vi "SERIAL_DecodeBinaryPacket.vi"(0 "navX DevRef":T1={"SerialPortRef"={"DevStatus"={"status"=FALSE, "code"=0, "source"=""}, "Serial Port Name"=""}, "Board Information"={"WhoAmI (50 | 0x32)"=0, "Board Revision"=0, "Firmware Major Version"=0, "Firmware Minor Version"=0, "NAVX_BOARD_CAPABILITY"={"OMNIMOUNT"=FALSE, "YAW_RESET"=FALSE, "VEL_AND_DISP"=FALSE}, "NAVX_BOARD_YAW_AXIS"={"BOARD_YAW_AXIS_UP"=FALSE, "BOARD_YAW_AXIS"=0}}, "Status"={"Update Rate Hz"=0, "Accelerometer Full-Scale Range"=0, "Gyro Full-Scale Range"=0, "NAVX_OP_STATUS"=0, "NAVX_CAL_STATUS"=0, "NAVX_SELFTEST_STATUS"=0, "NAVX_SENSOR_STATUS"={"MOVING"=FALSE, "YAW_STABLE"=FALSE, "MAG_DISTURBANCE"=FALSE, "ALTITUDE_VALID"=FALSE, "SEALEVEL_PRESS_SET"=FALSE, "FUSED_HEADING_VALID"=FALSE}}, "Offsets"={"Yaw"=0.0, "Quat W"=0.0, "Quat X"=0.0, "Quat Y"=0.0, "Quat Z"=0.0}, "Update Rate (4Hz-60Hz)"=50, "Nav6Mode (YPR)"=enum."YPR", "refnum name"="", "error"={"status"=FALSE, "code"=0, "source"=""}, "Loop VI Refnum"=refnum, "Serial Port"=enum."Onboard RS-232"} {"Status"."NAVX_OP_STATUS" items=["INITIALIZING", "SELFTEST_IN_PROGRESS", "ERROR", "IMU_AUTOCAL_IN_PROGRESS", "NORMAL"]; "Status"."NAVX_CAL_STATUS" items=["IMU_CAL_STATE_MASK"=3, "IMU_CAL_INPROGRESS"=0, "IMU_CAL_ACCUMULATE"=1, "IMU_CAL_COMPLETE"=2, "MAG_CAL_COMPLETE"=4, "BARO_CAL_COMPLETE"=8]}, 1 "PacketType":string, 2 "Buffer":string) -> (7 "navX DevRef":T1={"SerialPortRef"={"DevStatus"={"status"=FALSE, "code"=0, "source"=""}, "Serial Port Name"=""}, "Board Information"={"WhoAmI (50 | 0x32)"=0, "Board Revision"=0, "Firmware Major Version"=0, "Firmware Minor Version"=0, "NAVX_BOARD_CAPABILITY"={"OMNIMOUNT"=FALSE, "YAW_RESET"=FALSE, "VEL_AND_DISP"=FALSE}, "NAVX_BOARD_YAW_AXIS"={"BOARD_YAW_AXIS_UP"=FALSE, "BOARD_YAW_AXIS"=0}}, "Status"={"Update Rate Hz"=0, "Accelerometer Full-Scale Range"=0, "Gyro Full-Scale Range"=0, "NAVX_OP_STATUS"=0, "NAVX_CAL_STATUS"=0, "NAVX_SELFTEST_STATUS"=0, "NAVX_SENSOR_STATUS"={"MOVING"=FALSE, "YAW_STABLE"=FALSE, "MAG_DISTURBANCE"=FALSE, "ALTITUDE_VALID"=FALSE, "SEALEVEL_PRESS_SET"=FALSE, "FUSED_HEADING_VALID"=FALSE}}, "Offsets"={"Yaw"=0.0, "Quat W"=0.0, "Quat X"=0.0, "Quat Y"=0.0, "Quat Z"=0.0}, "Update Rate (4Hz-60Hz)"=50, "Nav6Mode (YPR)"=enum."YPR", "refnum name"="", "error"={"status"=FALSE, "code"=0, "source"=""}, "Loop VI Refnum"=refnum, "Serial Port"=enum."Onboard RS-232"} {"Status"."NAVX_OP_STATUS" items=["INITIALIZING", "SELFTEST_IN_PROGRESS", "ERROR", "IMU_AUTOCAL_IN_PROGRESS", "NORMAL"]; "Status"."NAVX_CAL_STATUS" items=["IMU_CAL_STATE_MASK"=3, "IMU_CAL_INPROGRESS"=0, "IMU_CAL_ACCUMULATE"=1, "IMU_CAL_COMPLETE"=2, "MAG_CAL_COMPLETE"=4, "BARO_CAL_COMPLETE"=8]})   [LabVIEW 2014, in "navX-MXP IMU.lvlib"]
uses:
  navX-MXP IMU.lvlib
  COMMON/TypeDefs/Data TypeDefs/navX Board Information.ctl
  COMMON/TypeDefs/Value TypeDefs/navX NAVX_BOARD_CAPABILITY.ctl
  COMMON/TypeDefs/Value TypeDefs/navX NAVX_BOARD_YAW_AXIS.ctl
  navX Serial DevRef.ctl
  <vilib>/Rock Robotics/WPI/SerialPort/WPI_SerialPortRef.ctl
  COMMON/TypeDefs/Data TypeDefs/navX Status Data.ctl
  COMMON/TypeDefs/Value TypeDefs/navX NAVX_OP_STATUS.ctl
  COMMON/TypeDefs/Value TypeDefs/navX NAVX_CAL_STATUS.ctl
  COMMON/TypeDefs/Value TypeDefs/navX NAVX_SENSOR_STATUS.ctl
  TypeDefs/navX Serial Mode.ctl
  IO/NI WPI/WPI_SerialPort_USB.ctl
  COMMON/TypeDefs/Data TypeDefs/navX YPRH Data.ctl
  COMMON/TypeDefs/Data TypeDefs/navX Vector Data.ctl
  COMMON/TypeDefs/Data TypeDefs/navX Quaternion Data.ctl
panel:
  out "Valid? 2":bool
  out "Valid?":bool
  in  "Board Information":T3
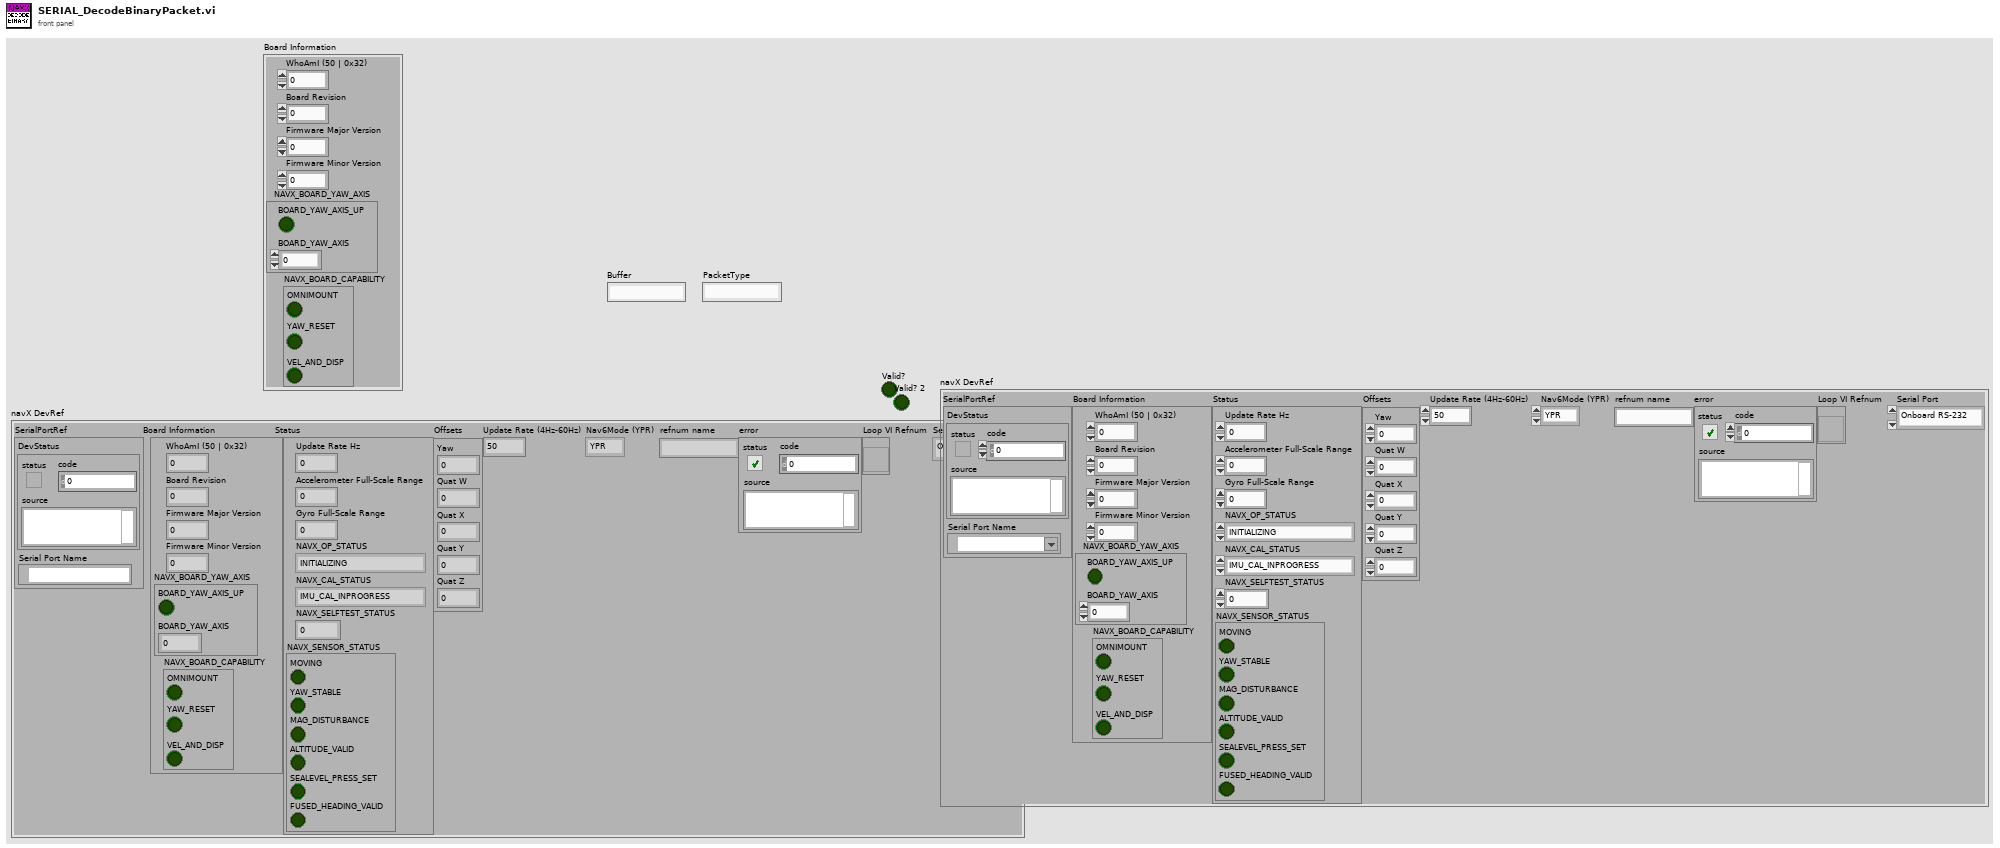
[diagram p1: front panel]
types:
  T1 = typedef "navX-MXP IMU.lvlib/navX Serial DevRef.ctl" = cluster{"SerialPortRef":T2, "Board Information":T3, "Status":T6, "Offsets":cluster{"Yaw":dbl, "Quat W":dbl, "Quat X":dbl, "Quat Y":dbl, "Quat Z":dbl}, "Update Rate (4Hz-60Hz)":u8, "Nav6Mode (YPR)":T10, "refnum name":string, "error":errorcluster, "Loop VI Refnum":refnum<vi>, "Serial Port":T11}
  T2 = typedef "WPI_SerialPortRef.ctl" = cluster{"DevStatus":errorcluster, "Serial Port Name":refnum<visa-resource-name>}
  T3 = typedef "navX-MXP IMU.lvlib/navX Board Information.ctl" = cluster{"WhoAmI (50 | 0x32)":u8, "Board Revision":u8, "Firmware Major Version":u8, "Firmware Minor Version":u8, "NAVX_BOARD_CAPABILITY":T4, "NAVX_BOARD_YAW_AXIS":T5}
  T4 = typedef "navX-MXP IMU.lvlib/navX NAVX_BOARD_CAPABILITY.ctl" = cluster{"OMNIMOUNT":bool, "YAW_RESET":bool, "VEL_AND_DISP":bool}
  T5 = typedef "navX-MXP IMU.lvlib/navX NAVX_BOARD_YAW_AXIS.ctl" = cluster{"BOARD_YAW_AXIS_UP":bool, "BOARD_YAW_AXIS":u8}
  T6 = typedef "navX-MXP IMU.lvlib/navX Status Data.ctl" = cluster{"Update Rate Hz":u8, "Accelerometer Full-Scale Range":u8, "Gyro Full-Scale Range":u16, "NAVX_OP_STATUS":T7, "NAVX_CAL_STATUS":T8, "NAVX_SELFTEST_STATUS":u8, "NAVX_SENSOR_STATUS":T9}
  T7 = typedef "navX-MXP IMU.lvlib/navX NAVX_OP_STATUS.ctl" = u8
  T8 = typedef "navX-MXP IMU.lvlib/navX NAVX_CAL_STATUS.ctl" = u8
  T9 = typedef "navX-MXP IMU.lvlib/navX NAVX_SENSOR_STATUS.ctl" = cluster{"MOVING":bool, "YAW_STABLE":bool, "MAG_DISTURBANCE":bool, "ALTITUDE_VALID":bool, "SEALEVEL_PRESS_SET":bool, "FUSED_HEADING_VALID":bool}
  T10 = typedef "navX-MXP IMU.lvlib/navX Serial Mode.ctl" = enum16{"YPR", "Gyro", "Quaternion", "AHRS", "AHRSPos"}
  T11 = typedef "navX-MXP IMU.lvlib/WPI_SerialPort_USB.ctl" = enum16{"Onboard RS-232", "MXP TTL", "USB"}
  T12 = typedef "navX-MXP IMU.lvlib/navX Quaternion Data.ctl" = cluster{"W":dbl, "X":dbl, "Y":dbl, "Z":dbl}
  T13 = typedef "navX-MXP IMU.lvlib/navX Vector Data.ctl" = cluster{"X":dbl, "Y":dbl, "Z":dbl}
  T14 = typedef "navX-MXP IMU.lvlib/navX YPRH Data.ctl" = cluster{"Yaw":dbl, "Pitch":dbl, "Roll":dbl, "Heading":dbl}
  T15 = cluster{"unsigned byte array[0]":u8, "unsigned byte array[1]":u8, "unsigned byte array[2]":u8, "unsigned byte array[3]":u8, "unsigned byte array[4]":u8, "unsigned byte array[5]":u8, "unsigned byte array[6]":u8, "unsigned byte array[7]":u8, "unsigned byte array[8]":u8}
  T16 = cluster{"[0]":u8, "[1]":u8, "[2]":u8, "[3]":u8, "[4]":u8, "[5]":u8, "[6]":u8, "[7]":u8, "[8]":u8}
  T17 = cluster{"Boolean array[0]":bool, "Boolean array[1]":bool, "Boolean array[2]":bool, "Boolean array[3]":bool, "Boolean array[4]":bool, "Boolean array[5]":bool}
  T18 = cluster{"[0]":dbl, "[1]":dbl, "[2]":dbl, "[3]":dbl}
  T19 = typedef "navX-MXP IMU.lvlib/navX AHRSPos Data.ctl" = cluster{"Quaternion":T12, "RawMag":T13, "CalMag":T13, "LinearAccel":T13, "Displacement":T13, "Velocity":T13, "Altitude":dbl, "FusedHeading":dbl, "MPU Temperature":dbl, "LastUpdateFPGATimestamp":dbl}
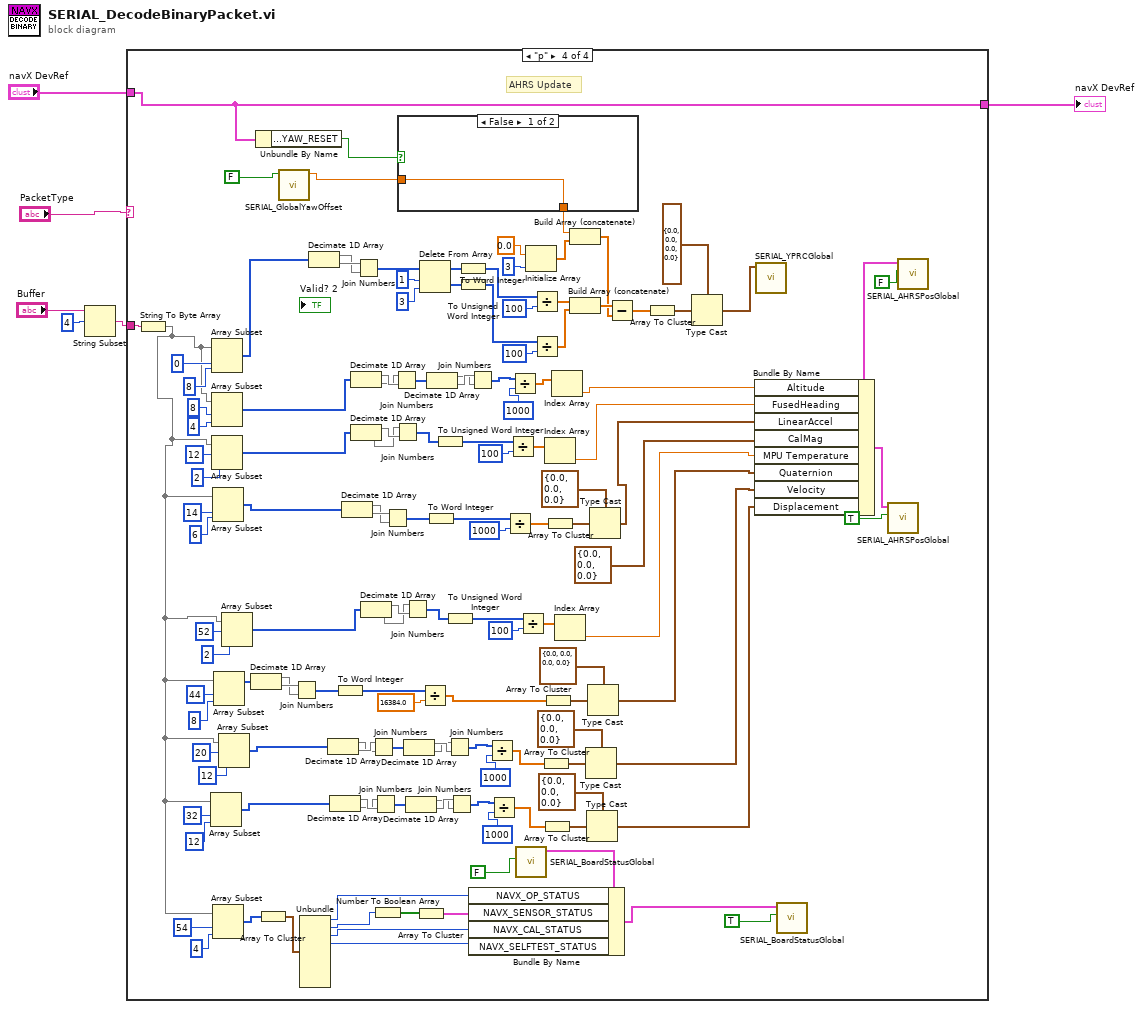
[diagram p0: block diagram]
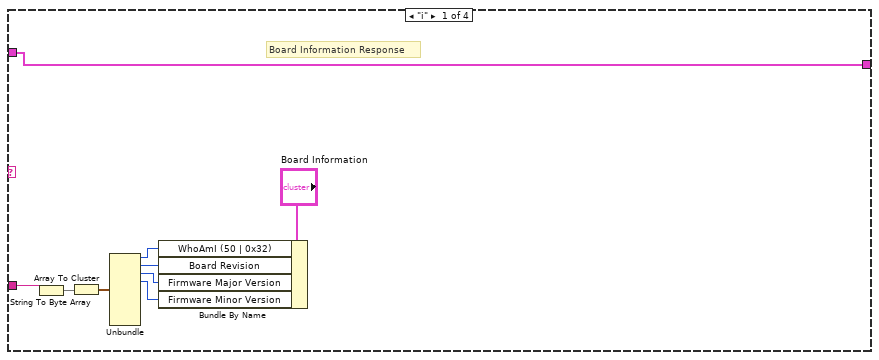
[diagram p2: hidden frame]
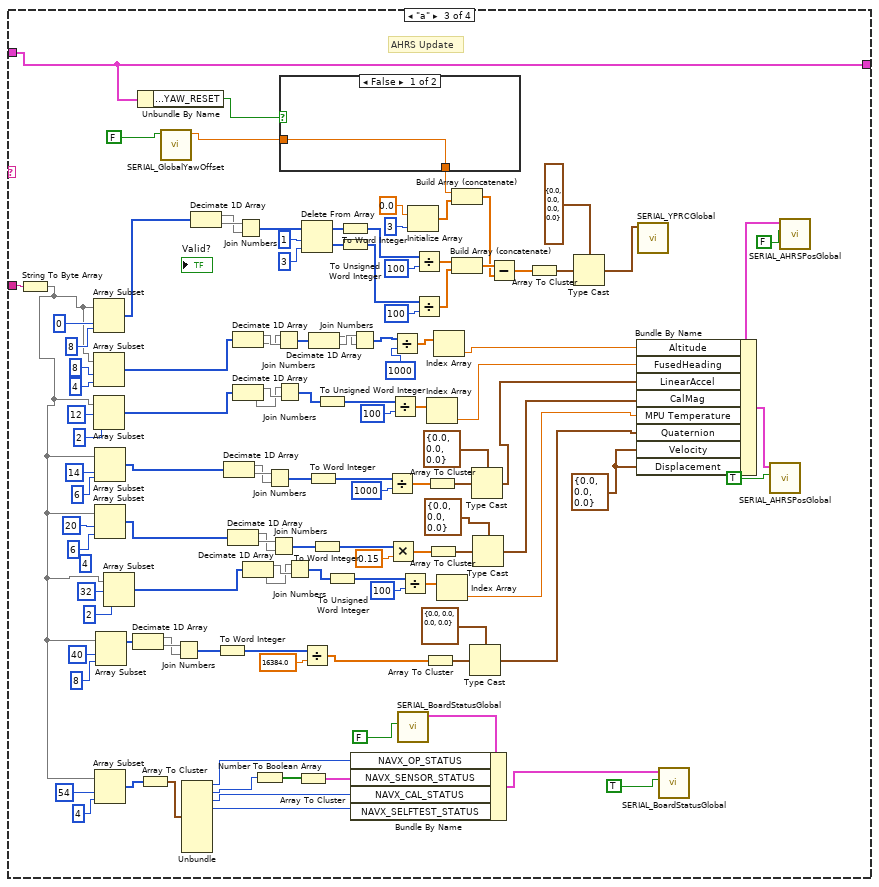
[diagram p4: hidden frame]
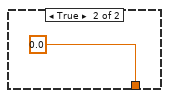
[diagram p5: hidden frame]
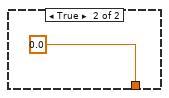
[diagram p6: hidden frame]
diagram:
  n1 = String Subset(string="Buffer", offset (0)=4) -> (substring=w4:string)  [unwired: 1 in]
  n2 = case shown="\"p\"" "PacketType" {
    tunnel: w4 -> [w9 _ w135 w272]
    tunnel: "navX DevRef" -> [w7 w16 w109 w246]
    tunnel: [w7 w16 w109 w246] -> w1
    frame "i" {
      # "Board Information Response"
      n3 = String To Byte Array(string=w9) -> (unsigned byte array=w8:u8[])
      n4 = Array To Cluster(array=w8) -> (cluster=w15:T15)
      n5 = Unbundle(w15) -> ("unsigned byte array[0]"=w13:u8, "unsigned byte array[1]"=w12:u8, "unsigned byte array[2]"=w11:u8, "unsigned byte array[3]"=w10:u8)  [unwired: 5 out]
      n6 = Bundle By Name(cluster="Board Information", "WhoAmI (50 | 0x32)"=w13, "Board Revision"=w12, "Firmware Major Version"=w11, "Firmware Minor Version"=w10) -> ()  [unwired: 1 out]
    }
    frame Default {
    }
    frame "a" {
      w18 = T13 {"X"=0.0, "Y"=0.0, "Z"=0.0} ("Vector")
      (unwired) 4
      # "AHRS Update"
      n7 = String To Byte Array(string=w135) -> (unsigned byte array=w22:u8[])
      n8 = Array Subset(array=w22, index=0, length=8) -> (w111:u8[])
      n9 = Array Subset(array=w22, index=8, length=4) -> (w89:u8[])
      n10 = Array Subset(array=w22, index=12, length=2) -> (w69:u8[])
      n11 = Array Subset(array=w22, index=14, length=6) -> (w56:u8[])
      n12 = Array Subset(array=w22, index=20, length=6) -> (w41:u8[])
      n13 = Array Subset(array=w22, index=54, length=4) -> (w100:u8[])
      n14 = Array Subset(array=w22, index=40, length=8) -> (w19:u8[])
      n15 = Array Subset(array=w22, index=32, length=2) -> (w40:u8[])
      n16 = Decimate 1D Array(w19) -> (w30:u8[], w31:u8[])
      n17 = Unbundle By Name(w109) -> ("Board Information.NAVX_BOARD_CAPABILITY.YAW_RESET"=w106:bool)
      n18 = Array To Cluster(array=w100) -> (cluster=w99:T16)
      n19 = call "SERIAL_GlobalYawOffset.vi"("Set"=FALSE) -> ("OutputYawOffset"=w107:dbl)  [unwired: 10 in]
      n20 = Join Numbers(hi=w31, lo=w30) -> ((hi.lo)=w29:u16[])
      n21 = Unbundle(w99) -> ("[0]"=w98:u8, "[1]"=w95:u8, "[2]"=w97:u8, "[3]"=w96:u8)  [unwired: 5 out]
      n22 = Decimate 1D Array(w111) -> (w133:u8[], w134:u8[])
      n23 = To Word Integer(number=w29) -> (16bit integer=w28:i16[])
      n24 = Decimate 1D Array(w56) -> (w64:u8[], w65:u8[])
      n25 = Decimate 1D Array(w41) -> (w52:u8[], w53:u8[])
      n26 = Decimate 1D Array(w89) -> (w88:u8[], w87:u8[])
      n27 = Decimate 1D Array(w69) -> (w68:u8[], w67:u8[])
      n28 = Join Numbers(hi=w134, lo=w133) -> ((hi.lo)=w131:u16[])
      n29 = Decimate 1D Array(w40) -> (w34:u8[], w33:u8[])
      n30 = Number To Boolean Array(number=w95) -> (Boolean array=w94:bool[])
      n31 = Join Numbers(hi=w65, lo=w64) -> ((hi.lo)=w63:u16[])
      n32 = Join Numbers(hi=w53, lo=w52) -> ((hi.lo)=w51:u16[])
      n33 = Join Numbers(hi=w87, lo=w88) -> ((hi.lo)=w86:u16[])
      n34 = Join Numbers(hi=w67, lo=w68) -> ((hi.lo)=w75:u16[])
      n35 = case shown="False" w106 {
        tunnel: w107 -> [w136 _]
        tunnel: [w136 0.0] -> w105
        frame False {
        }
        frame True {
        }
      }
      n36 = Join Numbers(hi=w33, lo=w34) -> ((hi.lo)=w35:u16[])
      n37 = Array To Cluster(array=w94) -> (cluster=w93:T17)
      n38 = Delete From Array(array=w131, length=1, index=3) -> (deleted portion=w127:u16[], array with subset deleted=w128:u16[])
      n39 = Divide(x=w28, y=16384.0) -> (x/y=w17:dbl[])
      n40 = To Word Integer(number=w63) -> (16bit integer=w62:i16[])
      n41 = Decimate 1D Array(w86) -> (w84:u16[], w85:u16[])
      n42 = To Word Integer(number=w51) -> (16bit integer=w50:i16[])
      n43 = To Unsigned Word Integer(number=w75) -> (unsigned 16bit integer=w74:u16[])
      n44 = To Unsigned Word Integer(number=w35) -> (unsigned 16bit integer=w36:u16[])
      n45 = To Word Integer(number=w128) -> (16bit integer=w114:i16[])
      n46 = To Unsigned Word Integer(number=w127) -> (unsigned 16bit integer=w126:u16[])
      n47 = Join Numbers(hi=w85, lo=w84) -> ((hi.lo)=w83:u32[])
      n48 = Divide(x=w62, y=1000) -> (x/y=w60:dbl[])
      n49 = Multiply(x=w50, y=0.15) -> (x*y=w49:dbl[])
      n50 = Divide(x=w74, y=100) -> (x/y=w72:dbl[])
      n51 = Divide(x=w83, y=i16 1000) -> (x/y=w81:dbl[])
      n52 = call "SERIAL_BoardStatusGlobal.vi"("Set"=FALSE) -> ("Status"=w101:T6)  [unwired: 9 in, 1 out]
      n53 = Bundle By Name(cluster=w101, "NAVX_OP_STATUS"=w98, "NAVX_SENSOR_STATUS"=w93, "NAVX_CAL_STATUS"=w97, "NAVX_SELFTEST_STATUS"=w96) -> (w91:T6)
      n54 = Divide(x=w36, y=100) -> (x/y=w38:dbl[])
      n55 = Initialize Array(0.0 ("element"), 3 ("dimension size")) -> (w120:dbl[])
      n56 = Divide(x=w114, y=i16 100) -> (x/y=w124:dbl[])
      n57 = Divide(x=w126, y=u16 100) -> (x/y=w123:dbl[])
      n58 = Array To Cluster(array=w17) -> (cluster=w26:T18)
      n59 = Index Array(array=w72) -> (element=w66:dbl)  [unwired: 1 in]
      n60 = Array To Cluster(array=w60) -> (cluster=w59:cluster{"[0]":dbl, "[1]":dbl, "[2]":dbl})
      n61 = Array To Cluster(array=w49) -> (cluster=w47:cluster{"[0]":dbl, "[1]":dbl, "[2]":dbl})
      n62 = Index Array(array=w81) -> (element=w76:dbl)  [unwired: 1 in]
      n63 = Index Array(array=w38) -> (element=w32:dbl)  [unwired: 1 in]
      n64 = Build Array (concatenate)(w105, w120) -> (w118:dbl[])
      n65 = Build Array (concatenate)(w124, w123) -> (w119:dbl[])
      n66 = Type Cast(type=T12 {"W"=0.0, "X"=0.0, "Y"=0.0, "Z"=0.0} ("Quaternion"), x=w26) -> (*(type *) &x=w24:T12)
      n67 = Type Cast(type=T13 {"X"=0.0, "Y"=0.0, "Z"=0.0} ("Vector"), x=w59) -> (*(type *) &x=w54:T13)
      n68 = Type Cast(type=T13 {"X"=0.0, "Y"=0.0, "Z"=0.0} ("Vector"), x=w47) -> (*(type *) &x=w45:T13)
      n69 = Subtract(x=w119, y=w118) -> (x-y=w117:dbl[])
      n70 = Array To Cluster(array=w117) -> (cluster=w116:T18)
      n71 = Type Cast(type=T14 {"Yaw"=0.0, "Pitch"=0.0, "Roll"=0.0, "Heading"=0.0} ("YPRH"), x=w116) -> (*(type *) &x=w110:T14)
      n72 = call "SERIAL_YPRCGlobal.vi"("YPRH"=w110) -> ()  [unwired: 9 in, 2 out]
      n73 = call "SERIAL_BoardStatusGlobal.vi"("Set"=TRUE, "Status"=w91) -> ()  [unwired: 8 in, 2 out]
      n74 = call "SERIAL_AHRSPosGlobal.vi"("Set"=FALSE) -> ("AHRSPos Data"=w79:T19)  [unwired: 10 in]
      n75 = Bundle By Name(cluster=w79, "Altitude"=w76, "FusedHeading"=w66, "LinearAccel"=w54, "CalMag"=w45, "MPU Temperature"=w32, "Quaternion"=w24, "Velocity"=w18, "Displacement"=w18) -> (w77:T19)
      n76 = call "SERIAL_AHRSPosGlobal.vi"("Set"=TRUE, "AHRSPos Data"=w77) -> ()  [unwired: 9 in, 1 out]
    }
    frame "p" {
      # "AHRS Update"
      n77 = String To Byte Array(string=w272) -> (unsigned byte array=w163:u8[])
      n78 = Array Subset(array=w163, index=32, length=12) -> (w147:u8[])
      n79 = Array Subset(array=w163, index=0, length=8) -> (w248:u8[])
      n80 = Array Subset(array=w163, index=8, length=4) -> (w226:u8[])
      n81 = Array Subset(array=w163, index=12, length=2) -> (w206:u8[])
      n82 = Array Subset(array=w163, index=14, length=6) -> (w193:u8[])
      n83 = Array Subset(array=w163, index=54, length=4) -> (w237:u8[])
      n84 = Array Subset(array=w163, index=44, length=8) -> (w169:u8[])
      n85 = Array Subset(array=w163, index=20, length=12) -> (w146:u8[])
      n86 = Array Subset(array=w163, index=52, length=2) -> (w189:u8[])
      n87 = Decimate 1D Array(w169) -> (w179:u8[], w180:u8[])
      n88 = Unbundle By Name(w246) -> ("Board Information.NAVX_BOARD_CAPABILITY.YAW_RESET"=w243:bool)
      n89 = Array To Cluster(array=w237) -> (cluster=w236:T16)
      n90 = call "SERIAL_GlobalYawOffset.vi"("Set"=FALSE) -> ("OutputYawOffset"=w244:dbl)  [unwired: 10 in]
      n91 = Join Numbers(hi=w180, lo=w179) -> ((hi.lo)=w178:u16[])
      n92 = Unbundle(w236) -> ("[0]"=w235:u8, "[1]"=w232:u8, "[2]"=w234:u8, "[3]"=w233:u8)  [unwired: 5 out]
      n93 = Decimate 1D Array(w248) -> (w270:u8[], w271:u8[])
      n94 = Decimate 1D Array(w146) -> (w155:u8[], w156:u8[])
      n95 = Decimate 1D Array(w147) -> (w154:u8[], w153:u8[])
      n96 = To Word Integer(number=w178) -> (16bit integer=w177:i16[])
      n97 = Decimate 1D Array(w193) -> (w201:u8[], w202:u8[])
      n98 = Decimate 1D Array(w226) -> (w225:u8[], w224:u8[])
      n99 = Decimate 1D Array(w206) -> (w205:u8[], w204:u8[])
      n100 = Join Numbers(hi=w271, lo=w270) -> ((hi.lo)=w268:u16[])
      n101 = Decimate 1D Array(w189) -> (w183:u8[], w182:u8[])
      n102 = Join Numbers(hi=w156, lo=w155) -> ((hi.lo)=w157:u16[])
      n103 = Join Numbers(hi=w153, lo=w154) -> ((hi.lo)=w152:u16[])
      n104 = Number To Boolean Array(number=w232) -> (Boolean array=w231:bool[])
      n105 = Join Numbers(hi=w202, lo=w201) -> ((hi.lo)=w200:u16[])
      n106 = Join Numbers(hi=w224, lo=w225) -> ((hi.lo)=w223:u16[])
      n107 = Join Numbers(hi=w204, lo=w205) -> ((hi.lo)=w212:u16[])
      n108 = case shown="False" w243 {
        tunnel: w244 -> [w273 _]
        tunnel: [w273 0.0] -> w242
        frame False {
        }
        frame True {
        }
      }
      n109 = Join Numbers(hi=w182, lo=w183) -> ((hi.lo)=w184:u16[])
      n110 = Decimate 1D Array(w157) -> (w159:u16[], w158:u16[])
      n111 = Decimate 1D Array(w152) -> (w150:u16[], w151:u16[])
      n112 = Array To Cluster(array=w231) -> (cluster=w230:T17)
      n113 = Delete From Array(array=w268, length=1, index=3) -> (deleted portion=w264:u16[], array with subset deleted=w265:u16[])
      n114 = Divide(x=w177, y=16384.0) -> (x/y=w168:dbl[])
      n115 = To Word Integer(number=w200) -> (16bit integer=w199:i16[])
      n116 = Decimate 1D Array(w223) -> (w221:u16[], w222:u16[])
      n117 = To Unsigned Word Integer(number=w212) -> (unsigned 16bit integer=w211:u16[])
      n118 = To Unsigned Word Integer(number=w184) -> (unsigned 16bit integer=w185:u16[])
      n119 = Join Numbers(hi=w158, lo=w159) -> ((hi.lo)=w160:u32[])
      n120 = Join Numbers(hi=w151, lo=w150) -> ((hi.lo)=w149:u32[])
      n121 = To Word Integer(number=w265) -> (16bit integer=w251:i16[])
      n122 = To Unsigned Word Integer(number=w264) -> (unsigned 16bit integer=w263:u16[])
      n123 = Join Numbers(hi=w222, lo=w221) -> ((hi.lo)=w220:u32[])
      n124 = Divide(x=w160, y=i16 1000) -> (x/y=w144:dbl[])
      n125 = Divide(x=w149, y=i16 1000) -> (x/y=w139:dbl[])
      n126 = Divide(x=w199, y=1000) -> (x/y=w197:dbl[])
      n127 = Divide(x=w211, y=100) -> (x/y=w209:dbl[])
      n128 = Divide(x=w220, y=i16 1000) -> (x/y=w218:dbl[])
      n129 = call "SERIAL_BoardStatusGlobal.vi"("Set"=FALSE) -> ("Status"=w238:T6)  [unwired: 9 in, 1 out]
      n130 = Bundle By Name(cluster=w238, "NAVX_OP_STATUS"=w235, "NAVX_SENSOR_STATUS"=w230, "NAVX_CAL_STATUS"=w234, "NAVX_SELFTEST_STATUS"=w233) -> (w228:T6)
      n131 = Divide(x=w185, y=100) -> (x/y=w187:dbl[])
      n132 = Initialize Array(0.0 ("element"), 3 ("dimension size")) -> (w257:dbl[])
      n133 = Divide(x=w251, y=i16 100) -> (x/y=w261:dbl[])
      n134 = Divide(x=w263, y=u16 100) -> (x/y=w260:dbl[])
      n135 = Array To Cluster(array=w144) -> (cluster=w145:cluster{"[0]":dbl, "[1]":dbl, "[2]":dbl})
      n136 = Array To Cluster(array=w139) -> (cluster=w140:cluster{"[0]":dbl, "[1]":dbl, "[2]":dbl})
      n137 = Array To Cluster(array=w168) -> (cluster=w175:T18)
      n138 = Index Array(array=w209) -> (element=w203:dbl)  [unwired: 1 in]
      n139 = Array To Cluster(array=w197) -> (cluster=w196:cluster{"[0]":dbl, "[1]":dbl, "[2]":dbl})
      n140 = Index Array(array=w218) -> (element=w213:dbl)  [unwired: 1 in]
      n141 = Index Array(array=w187) -> (element=w181:dbl)  [unwired: 1 in]
      n142 = Build Array (concatenate)(w242, w257) -> (w255:dbl[])
      n143 = Build Array (concatenate)(w261, w260) -> (w256:dbl[])
      n144 = Type Cast(type=T13 {"X"=0.0, "Y"=0.0, "Z"=0.0} ("Vector"), x=w145) -> (*(type *) &x=w142:T13)
      n145 = Type Cast(type=T13 {"X"=0.0, "Y"=0.0, "Z"=0.0} ("Vector"), x=w140) -> (*(type *) &x=w138:T13)
      n146 = Type Cast(type=T12 {"W"=0.0, "X"=0.0, "Y"=0.0, "Z"=0.0} ("Quaternion"), x=w175) -> (*(type *) &x=w173:T12)
      n147 = Type Cast(type=T13 {"X"=0.0, "Y"=0.0, "Z"=0.0} ("Vector"), x=w196) -> (*(type *) &x=w191:T13)
      n148 = Subtract(x=w256, y=w255) -> (x-y=w254:dbl[])
      n149 = Array To Cluster(array=w254) -> (cluster=w253:T18)
      n150 = Type Cast(type=T14 {"Yaw"=0.0, "Pitch"=0.0, "Roll"=0.0, "Heading"=0.0} ("YPRH"), x=w253) -> (*(type *) &x=w247:T14)
      n151 = call "SERIAL_YPRCGlobal.vi"("YPRH"=w247) -> ()  [unwired: 9 in, 2 out]
      n152 = call "SERIAL_BoardStatusGlobal.vi"("Set"=TRUE, "Status"=w228) -> ()  [unwired: 8 in, 2 out]
      n153 = call "SERIAL_AHRSPosGlobal.vi"("Set"=FALSE) -> ("AHRSPos Data"=w216:T19)  [unwired: 10 in]
      n154 = Bundle By Name(cluster=w216, "Altitude"=w213, "FusedHeading"=w203, "LinearAccel"=w191, "CalMag"=T13 {"X"=0.0, "Y"=0.0, "Z"=0.0} ("Vector"), "MPU Temperature"=w181, "Quaternion"=w173, "Velocity"=w142, "Displacement"=w138) -> (w214:T19)
      n155 = call "SERIAL_AHRSPosGlobal.vi"("Set"=TRUE, "AHRSPos Data"=w214) -> ()  [unwired: 9 in, 1 out]
    }
  }
  "navX DevRef" <- w1
